vi "Return Messages.vi"(1 "Nombre à convertir":u16) -> (0 "Message Axe":string)   [LabVIEW 2013]
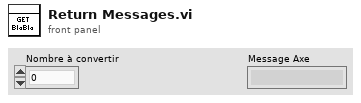
[diagram p1: front panel]
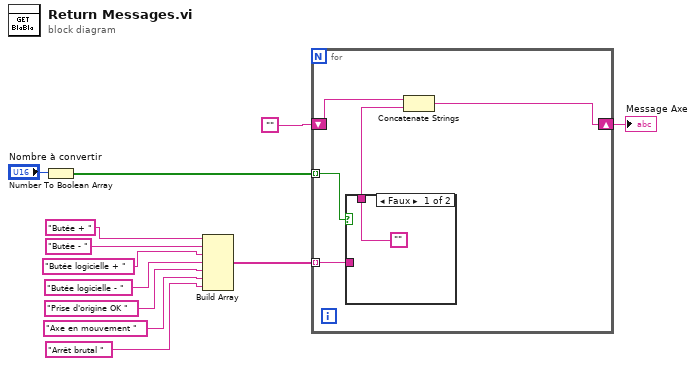
[diagram p0: block diagram]
diagram:
  n1 = Number To Boolean Array(number="Nombre à convertir") -> (Boolean array=w1:bool[])
  n2 = Build Array("Butée + ", "Butée - ", "Butée logicielle + ", "Butée logicielle - ", "Prise d'origine OK ", "Axe en mouvement ", "Arrêt brutal ") -> (w5:string[])
  n3 = for {
    tunnel: w5 -> [w17] mode=indexing
    shift-right: [w14] -> w2
    shift-left: "" -> [w16]
    tunnel: w1 -> [w13] mode=indexing
    n4 = case shown="Faux" w13 {
      tunnel: w17 -> [_ w19]
      tunnel: ["" w19] -> w15
      frame False {
      }
      frame True {
      }
    }
    n5 = Concatenate Strings(w16, w15) -> (w14:string)
  }
  "Message Axe" <- w2
